vi "delete.vi"(8 "error in (no error)":errorcluster, 10 "key chain":string[](array[string]), 11 "Map in":refnum<class "Map.lvclass">) -> (0 "error out":errorcluster, 3 "Map out":refnum<class "Map.lvclass">)   [LabVIEW 2010, in "Map.lvclass"]
doc: "This method deletes a specific node from a nested or non-nested map. The position is specified by the key array. \nFor a nested map, the key array contains all keys from root down to the desired position. For a non-nested map, simply provide an array with a single key value."
uses:
  Map.lvclass
  Map.lvclass/Map.ctl
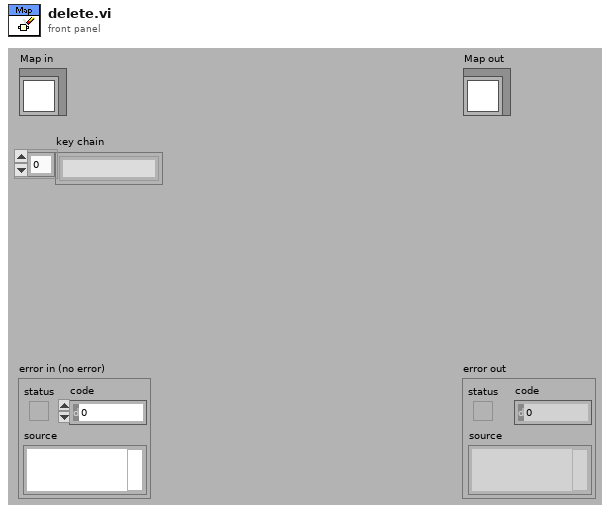
[diagram p1: front panel]
types:
  T1 = typedef "Map.lvclass/element_cluster.ctl" = cluster{"key":string, "value":variant}
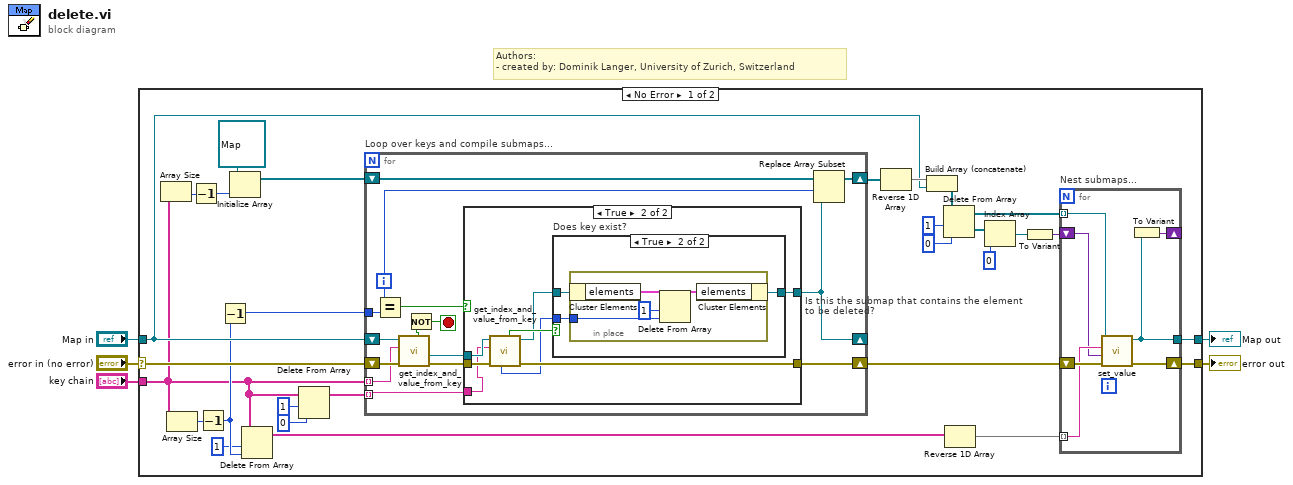
[diagram p0: block diagram]
diagram:
  # "Authors: \n- created by: Dominik Langer, University of Zurich, Switzerland"
  n1 = case shown="No Error" "error in (no error)" {
    selector: "error in (no error)" -> [w34 w76]
    tunnel: [w8 w76] -> w4
    tunnel: [w9 w75] -> w2
    tunnel: "Map in" -> [w27 w75]
    tunnel: "key chain" -> [w17 _]
    frame No Error {
      n2 = Array Size(array=w17) -> (size(s)=w32:i32)
      n3 = Array Size(array=w17) -> (size(s)=w25:i32)
      n4 = Decrement(x=w32) -> (x-1=w31:i32)
      n5 = Decrement(x=w25) -> (x-1=w24:i32)
      n6 = Decrement(x=w24) -> (x-1=w23:i32)
      n7 = Initialize Array(refnum<class "Map.lvclass"> refnum ("Map.lvclass"), w31) -> (w30:refnum<class "Map.lvclass">[])
      n8 = Delete From Array(array=w17, length=1, index=w24) -> (array with subset deleted=w20:string[])  [unwired: 1 out]
      n9 = Delete From Array(array=w17, length=1, index=0) -> (array with subset deleted=w16:string[])  [unwired: 1 out]
      n10 = for "Loop over keys and compile submaps..." {
        tunnel: w17 -> [w54] mode=indexing
        shift-right: [w51] -> w26
        shift-left: w34 -> [w56]
        shift-right: [w42] -> _
        shift-left: w27 -> [w55]
        shift-right: [w45] -> w28
        shift-left: w30 -> [w44]
        tunnel: w23 -> [w49]
        tunnel: w16 -> [w43] mode=indexing
        i -> [w46]
        stop <- w53 stop-if-true
        n11 = Equal?(x=w46, y=w49) -> (x = y?=w48:bool)
        n12 = call "get_index_and_value_from_key.vi"("error in (no error)"=w56, "key"=w54, "Map.lvclass in"=w55) -> ("error out"=w52:errorcluster, "submap"=w50:refnum<class "Map.lvclass">, "key exists?"=w47:bool)  [unwired: 6 out]
        n13 = Not(x=w47) -> (.not. x?=w53:bool)
        n14 = case "Is this the submap that contains the element to be deleted?" shown="True" w48 {
          tunnel: w52 -> [w58 w65]
          tunnel: [w58 w64] -> w51
          tunnel: w50 -> [w57 w63]
          tunnel: [w57 w66] -> w42
          tunnel: w43 -> [_ w59]
          frame False {
          }
          frame True {
            n15 = call "get_index_and_value_from_key.vi"("error in (no error)"=w65, "key"=w59, "Map.lvclass in"=w63) -> ("error out"=w64:errorcluster, "Map.lvclass out"=w60:refnum<class "Map.lvclass">, "key exists?"=w62:bool, "index"=w61:i32)  [unwired: 5 out]
            n16 = case "Does key exist?" shown="True" w62 {
              tunnel: w60 -> [w67 w70]
              tunnel: w61 -> [_ w69]
              tunnel: [w67 w68] -> w66
              frame False {
              }
              frame True {
                n17 = in-place {
                  in-place-border: w69 -> [w73]
                  n18 = in-place-cluster #1(w70) -> ("elements"=w74:T1[])
                  n19 = Delete From Array(array=w74, length=1, index=w73) -> (array with subset deleted=w72:T1[])  [unwired: 1 out]
                  n20 = in-place-cluster #1("elements"=w72) -> (w68:refnum<class "Map.lvclass">)
                }
              }
            }
          }
        }
        n21 = Replace Array Subset(array=w44, new element=w42, index=w46) -> (w45:refnum<class "Map.lvclass">[])
      }
      n22 = Reverse 1D Array(array=w28) -> (reversed array=w29:refnum<class "Map.lvclass">[])
      n23 = Build Array (concatenate)(w29, w27) -> (w7:refnum<class "Map.lvclass">[])
      n24 = Delete From Array(array=w7, length=1, index=0) -> (deleted portion=w13:refnum<class "Map.lvclass">[], array with subset deleted=w14:refnum<class "Map.lvclass">[])
      n25 = Reverse 1D Array(array=w20) -> (reversed array=w22:string[])
      n26 = Index Array(array=w13, index=0) -> (element=w11:refnum<class "Map.lvclass">)
      n27 = To Variant(anything=w11) -> (Variant=w10:variant)
      n28 = for "Nest submaps..." {
        shift-right: [w39] -> w8
        shift-left: w26 -> [w41]
        tunnel: w22 -> [w40] mode=indexing
        shift-right: [w37] -> _
        shift-left: w10 -> [w36]
        tunnel: w14 -> [w38] mode=indexing
        tunnel: [w35] -> w9
        n29 = call "set_value.vi"("error in (no error)"=w41, "value"=w36, "key"=w40, "Map.lvclass in"=w38) -> ("error out"=w39:errorcluster, "Map.lvclass out"=w35:refnum<class "Map.lvclass">)  [unwired: 6 out]
        n30 = To Variant(anything=w35) -> (Variant=w37:variant)
      }
    }
    frame Error {
    }
  }
  "error out" <- w4
  "Map out" <- w2
